vi "Triangles to vertices (without duplicates).vi"(1 "Triangles":T1[](array[typedef])) -> (0 "Vertices (without duplicates)":sgl[][](array[numeric]))   [LabVIEW 2014]
uses:
  Typedefs/Triangle.ctl
  Dot product.vi
panel:
  # "PN 21/03/2015"
  # "Vertices"
  # "Edges"
  # "Unit normal"
  # "Edge unit normals"
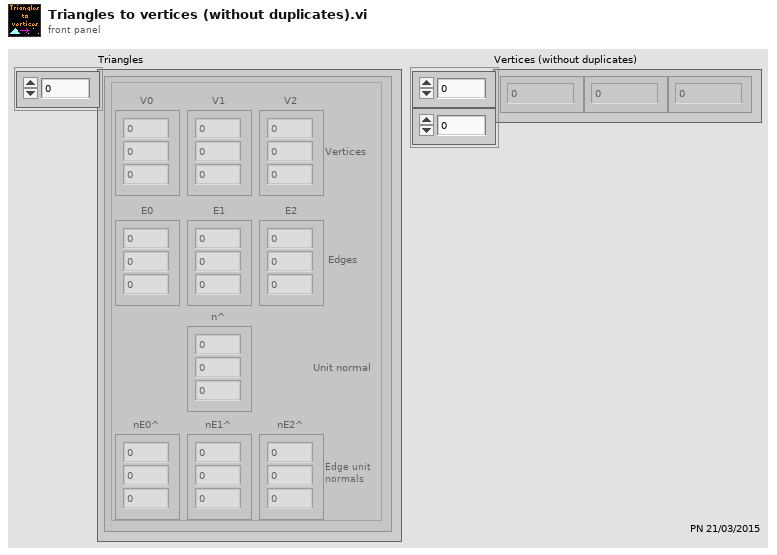
[diagram p1: front panel]
types:
  T1 = typedef "Triangle.ctl" = cluster{"V0":sgl[], "V1":sgl[], "V2":sgl[], "E0":sgl[], "E1":sgl[], "E2":sgl[], "n^":sgl[], "nE0^":sgl[], "nE1^":sgl[], "nE2^":sgl[]}
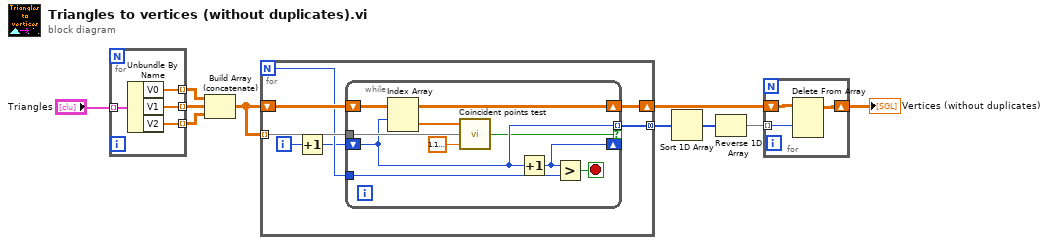
[diagram p0: block diagram]
diagram:
  n1 = for {
    tunnel: "Triangles" -> [w14] mode=indexing
    tunnel: [w13] -> w9 mode=indexing
    tunnel: [w12] -> w8 mode=indexing
    tunnel: [w11] -> w7 mode=indexing
    n2 = Unbundle By Name(w14) -> ("V0"=w13:sgl[], "V1"=w12:sgl[], "V2"=w11:sgl[])
  }
  n3 = Build Array (concatenate)(w9, w8, w7) -> (w6:sgl[][])
  n4 = for {
    N -> [w17]
    shift-right: [w20] -> w4
    shift-left: w6 -> [w20]
    tunnel: w6 -> [w19] mode=indexing
    tunnel: [w15] -> w5 mode=concatenating
    i -> [w18]
    n5 = Increment(x=w18) -> (x+1=w16:i32)
    n6 = while {
      tunnel: w19 -> [w29]
      shift-right: [w25] -> _
      shift-left: w16 -> [w22]
      shift-right: [w27] -> _
      shift-left: w20 -> [w27]
      tunnel: w17 -> [w24]
      tunnel: [w22] -> w15 mode=indexing if=w21
      stop <- w26 stop-if-true
      n7 = Index Array(array=w27, index (row)=w22) -> (element=w28:sgl[])  [unwired: 1 in]
      n8 = call "Coincident points test.vi"("epsilon"=sgl 1.1920929e-07, "Point 2"=w29, "Point 1"=w28) -> ("Points are coincident"=w21:bool)
      n9 = Increment(x=w22) -> (x+1=w25:i32)
      n10 = Greater?(x=w25, y=w24) -> (0:w26:bool)
    }
  }
  n11 = Sort 1D Array(array=w5) -> (sorted array=w3:i32[])
  n12 = Reverse 1D Array(array=w3) -> (reversed array=w2:i32[])
  n13 = for {
    tunnel: w2 -> [w31] mode=indexing
    shift-right: [w30] -> w1
    shift-left: w4 -> [w32]
    n14 = Delete From Array(array=w32, index (row)=w31) -> (array with subset deleted=w30:sgl[][])  [unwired: 2 in, 1 out]
  }
  "Vertices (without duplicates)" <- w1
